vi "editDialog.vi"(0 "reference":refnum<class "CallEdge.lvclass">, 5 "error in (no error)":errorcluster) -> (14 "reference out":refnum<class "CallEdge.lvclass">, 15 "cancel":bool, 19 "error out":errorcluster)   [LabVIEW 2016, in "CallEdge.lvclass"]
doc: "Edit Dialog"
uses:
  <resource>/Framework/Providers/Open_GDS/UML/CallEdge_class/CallEdge.lvclass
  C:/Program Files (x86)/National Instruments/LabVIEW 2016/resource/Framework/Providers/Open_GDS/UML/SegmentedLineEdge_class/SegmentedLineEdge.lvclass
  <resource>/Framework/Providers/Open_GDS/UML/ContextHelp/ContextHelp_HelpTexts.ctl
  <resource>/Framework/Providers/Open_GDS/UML/SegmentedLineEdge_class/SegmentedLineEdge.lvclass
panel:
  in  "OK Button":bool
  in  "Cancel Button":bool
  in  "Help":bool
  in  "Call text":string
  in  "Is signal":bool
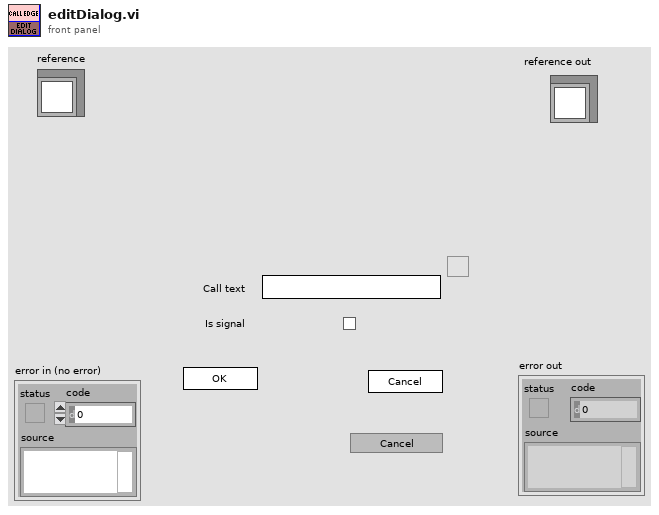
[diagram p1: front panel]
types:
  T1 = typedef "ContextHelp_HelpTexts.ctl" = enum16{"None(Hide)", "Default", "Help", "Welcome", "GettingStarted", "ClassDiagram_Help", "SequenceDiagram_Help", "UseCaseDiagram_Help", "BSelect", "BClass", "BInterface", "BPackage", "BNote", "BDependency", "BInheritance", "BInterfaceImplementation", "BAssociation", "BAggregation", "BCompAggregation", "BNoteConnector", "BObject", "BActionBar", "BCall", "BSystem", "BActor", "BUseCase", "BGeneralization", "BIncludes", "BExtends", "BUseCaseDiagramAssociation", "ClassRelationshipEdge editDialog_Bent Style", "ClassRelationshipEdge editDialog_RelationType", "ClassRelationshipEdge editDialog_Reverse association", "ClassRelationshipEdge editDialog_Start label", "ClassRelationshipEdge editDialog_Middle label", "ClassRelationshipEdge editDialog_End label", "UMLEditor reversedEngineering_Pathes", "ReversedEngineering StateReverseDialog_Help", "ReversedEngineering StateQueuedSettings_Help", "UMLEditor reversedEngineering_AddTopVIs", "UMLEditor reversedEngineering_AddClasses", "UMLEditor reversedEngineering_AddDirs", "UMLEditor reversedEngineering_Recursively", "UMLEditor reversedEngineering_Remove", "UMLEditor reversedEngineering_ClearList", "UMLEditor reversedEngineering_HideSubAss", "UMLEditor reversedEngineering_CreateTypes", "UMLEditor reversedEngineering_OnlyInheritance", "UMLEditor reversedEngineering_CreateApplication", "UMLEditor reversedEngineering_OK", "UMLEditor reversedEngineering_Cancel", "UMLEditor reversedEngineering_Help", "UMLEditor createWizardScriptFile_ScriptfilePath", "UMLEditor createWizardScriptFile_ClassPath", "UMLEditor createWizardScriptFile_Use", "UMLEditor createWizardScriptFile_PrivateDirName", "UMLEditor createWizardScriptFile_DirAppend", "UMLEditor createWizardScriptFile_Separator Character", "UMLEditor createWizardScriptFile_OK", "UMLEditor createWizardScriptFile_Cancel", "UMLEditor createWizardScriptFile_Help", "ClassNode editDialog_Class Name", "InterfaceNode editDialog_Class Name", "ClassNode editDialog_Attribute", "ClassNode editDialog_Methods", "InterfaceNode editDialog_Methods", "ClassNode editDialog_connection", "InterfaceNode editDialog_connection", "ClassNode editDialog_StereoType", "ClassNode editDialog_ShowAttrib", "ClassNode editDialog_ShowMethods", "ClassNode editDialog_ClassPath", "ClassNode editDialog_AddAttribute", "ClassNode editDialog_AddMethod", "InterfaceNode editDialog_AddMethod", "ClassNode AttributeGuide_AttributeName", "ClassNode AttributeGuide_Array?", "ClassNode AttributeGuide_Data Type", "ClassNode AttributeGuide_RefName", "ClassNode AttributeGuide_Preview", "ClassNode AttributeGuide_OK", "ClassNode AttributeGuide_Cancel", "ClassNode MethodGuide_Visibility", "ClassNode MethodGuide_Method Name", "ClassNode MethodGuide_Preview", "ClassNode MethodGuide_OK", "ClassNode MethodGuide_Cancel", "CallNode EditCallProperties_AllButtons", "ObjectNode EditObjectlProperties_AllButtons", "ActorNode EditActorProperties_AllButtons", "UseCaseRelationshipNode EditUseCaselProperties_AllButtons", "UseCaseNode EditUseCaselProperties_AllButtons", "SystemNode EditSystemProperties_AllButtons", "ReversedEngineering UpdateAttributes_AllButtons", "StateNode editDialog_AllButtons", "StateTransition editDialog_AllButtons", "ArrangeNodes Main_Picture", "ArrangeNodes Main_Zoom", "ArrangeNodes Main_Auto Zoom", "ArrangeNodes Main_shorten", "ArrangeNodes Main_Min Length", "ArrangeNodes Main_Max Length", "ArrangeNodes Main_increase", "ArrangeNodes Main_decrease", "ArrangeNodes Main_Shake", "ArrangeNodes Main", "BState", "BInitialState", "BFinalState", "BStateTransition", "StateDiagram_Help", "StateDiagram_PropertiesAllButtons", "ReversedEngineering StateReverseDialog_ClearStates", "ReversedEngineering StateReverseDialog_UseQueuedStateMachines", "ReversedEngineering StateReverseDialog_QueuedSettings", "ReversedEngineering StateReverseDialog_SearchForVIs", "ReversedEngineering StateReverseDialog_SearchCriteria", "OptionsDialog_ClassBasePath", "OptionsDialog_VIPath", "OptionsDialog_ApplicationPath", "OptionsDialog_WizDir", "OptionsDialog_IniFilePath", "OptionsDialog_DefineColors", "OptionsDialog_Help", "OptionsDialog_CreateTypes", "ClassRelationshipEdge editDialog_SplitWire"}
  T2 = typedef "CallEdge.lvclass/ObjectAttributes.ctl" = cluster{"signal":bool}
  T3 = typedef "SegmentedLineEdge.lvclass/ObjectAttributes.ctl" = cluster{"lineStyle":refnum<class "LineStyle.lvclass">, "startArrowHead":refnum<class "ArrowHead.lvclass">, "endArrowHead":refnum<class "ArrowHead.lvclass">, "startLabel":string, "midLabel":string, "endLabel":string, "MidLabelOffset":T4, "SplitWire":bool}
  T4 = typedef "Point Point2D.ctl" = cluster{"x":dbl, "y":dbl}
  T5 = typedef "ContextHelp_ShowType.ctl" = cluster{"Header":string, "Picture":picture, "Text":string}
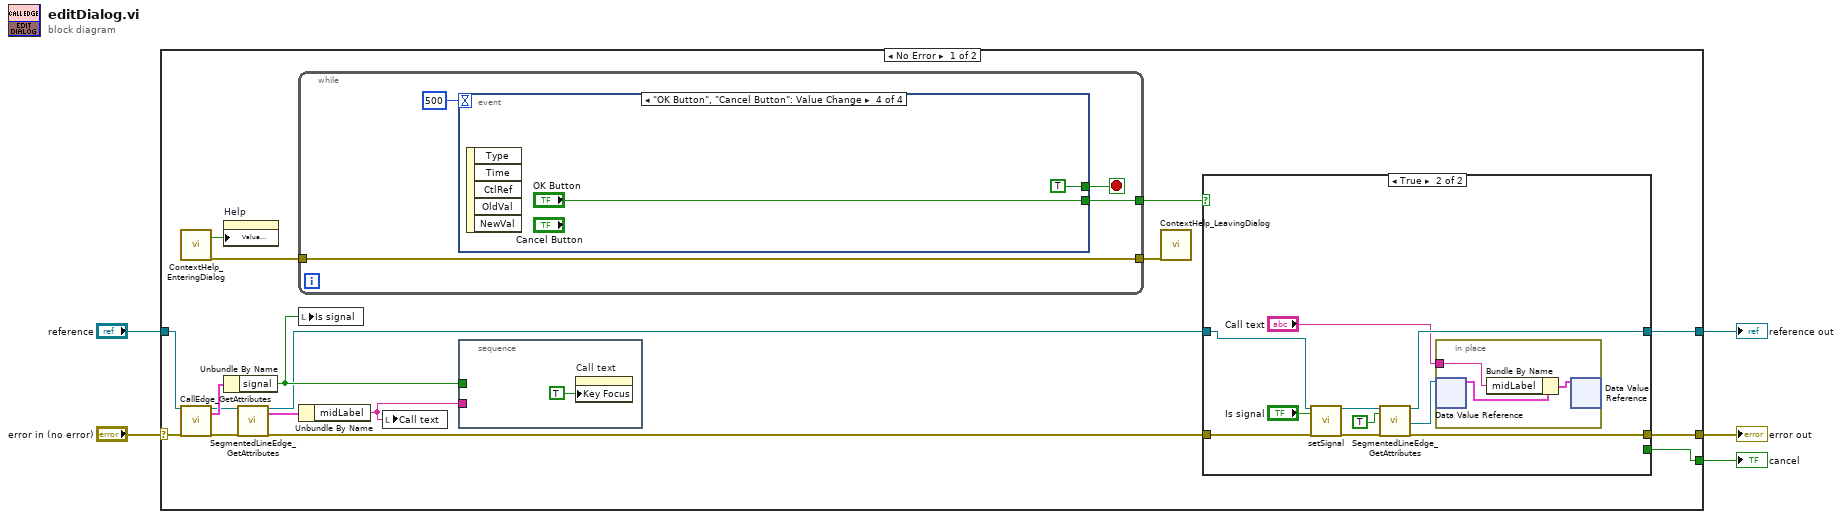
[diagram p0: block diagram]
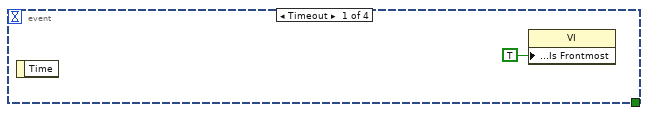
[diagram p2: hidden frame]
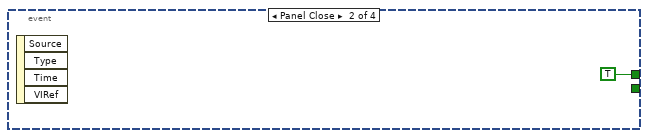
[diagram p3: hidden frame]
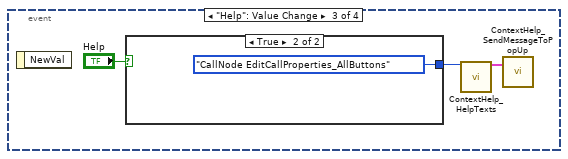
[diagram p4: hidden frame]
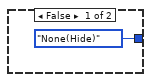
[diagram p5: hidden frame]
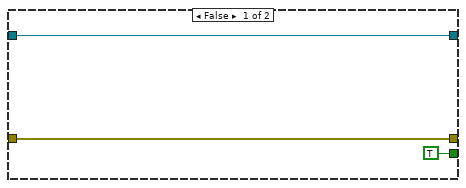
[diagram p6: hidden frame]
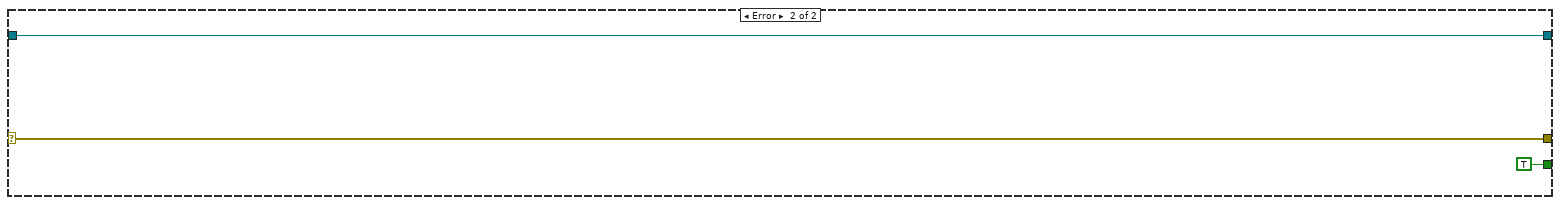
[diagram p7: hidden frame]
diagram:
  n1 = case shown="No Error" "error in (no error)" {
    selector: "error in (no error)" -> [w19 w54]
    tunnel: "reference" -> [w20 w55]
    tunnel: [w22 w54] -> w3
    tunnel: [w21 w55] -> w2
    tunnel: [w18 TRUE ("Key Focus")] -> w1
    frame No Error {
      n2 = call <resource>:"ContextHelp_EnteringDialog.vi"() -> ("HelpStatus"=w13:bool, "error out"=w14:errorcluster)  [unwired: 3 in, 15 out]
      n3 = call <resource>:"CallEdge_GetAttributes.vi"("reference in"=w20, "error in (no error)"=w19) -> ("reference out"=w10:refnum<class "CallEdge.lvclass">, "Data"=w11:T2, "error out"=w9:errorcluster)  [unwired: 1 in, 14 out]
      n4 = property on="Help" class="Bool (strict)"("Value (Signaling)"=w13) -> ()  [unwired: 2 in, 2 out]
      n5 = Unbundle By Name(w11) -> ("signal"=w17:bool)
      n6 = call <resource>:"SegmentedLineEdge_GetAttributes.vi"("reference in"=w10, "error in (no error)"=w9) -> ("reference out"=w7:refnum<class "CallEdge.lvclass">, "Data"=w6:T3, "error out"=w8:errorcluster)  [unwired: 14 in, 1 out]
      n7 = while {
        tunnel: [w26] -> w12
        tunnel: [w24] -> w15
        tunnel: w14 -> [w24]
        stop <- w25 stop-if-true
        n8 = event shown="[3] \"OK Button\", \"Cancel Button\": Value Change" {
          selector: _ -> [_ _ _ _]
          dyn-events: _ -> [_ _ _ _]
          timeout: 500 -> [_ _ _ _]
          tunnel: [_ _ _ "OK Button"] -> w26
          tunnel: [_ TRUE _ TRUE] -> w25
          event Timeout {
            n9 = event-data() -> ()  [unwired: 2 out]
            n10 = property class="VI"("Front Panel Window:Is Frontmost"=TRUE) -> ()  [unwired: 2 in, 2 out]
          }
          event Panel Close {
            n11 = event-data() -> ()  [unwired: 5 out]
          }
          event "Help": Value Change {
            n12 = event-data() -> ()  [unwired: 2 out]
            n13 = case shown="True" "Help" {
              tunnel: [ContextHelp_HelpTexts."None(Hide)" ("HelpText") ContextHelp_HelpTexts."CallNode EditCallProperties_AllButtons" ("HelpText")] -> w30
              frame False {
              }
              frame True {
              }
            }
            n14 = call <resource>:"ContextHelp_HelpTexts.vi"("HelpText (enum or string)"=w30) -> ("HelpOut"=w31:T5)  [unwired: 18 out]
            n15 = call <resource>:"ContextHelp_SendMessageToPopUp.vi"("PopUpMessage"=w31) -> ()  [unwired: 2 in, 17 out]
          }
          event "OK Button", "Cancel Button": Value Change {
            n16 = event-data() -> ()  [unwired: 6 out]
          }
        }
      }
      n17 = local write "Is signal"(w17) -> ()
      n18 = Unbundle By Name(w6) -> ("midLabel"=w16:string)
      n19 = local write "Call text"(w16) -> ()
      n20 = stacked-sequence {
        tunnel: w17 -> [_]
        tunnel: w16 -> [_]
        frame #0 {
          n21 = property on="Call text" class="Str"("Key Focus"=TRUE) -> ()  [unwired: 2 in, 2 out]
        }
      }
      n22 = call <resource>:"ContextHelp_LeavingDialog.vi"("error in (no error)"=w15) -> ()  [unwired: 2 in, 17 out]
      n23 = case shown="True" w12 {
        tunnel: [w36 w48] -> w22
        tunnel: [w38 w47] -> w21
        tunnel: w7 -> [w38 w44]
        tunnel: [TRUE ("Key Focus") _] -> w18
        tunnel: w8 -> [w36 w43]
        frame False {
        }
        frame True {
          n24 = call-dynamic "setSignal.vi"("reference"=w44, "signal"="Is signal", "error in (no error)"=w43) -> ("reference out"=w46:refnum<class "CallEdge.lvclass">, "error out"=w45:errorcluster)  [unwired: 15 out]
          n25 = call <resource>:"SegmentedLineEdge_GetAttributes.vi"("reference in"=w46, "OnlyGetDvrReference(False)"=TRUE, "error in (no error)"=w45) -> ("reference out"=w47:refnum<class "CallEdge.lvclass">, "DataRef"=w40:refnum<data-value>, "error out"=w48:errorcluster)  [unwired: 13 in, 1 out]
          n26 = in-place {
            in-place-border: "Call text" -> [w50]
            n27 = in-place-dvr #1(w40) -> (w51:T3)  [unwired: 1 out]
            n28 = Bundle By Name(cluster=w51, "midLabel"=w50) -> (w49:T3)
            n29 = in-place-dvr #1(w49) -> ()  [unwired: 2 out]
          }
        }
      }
    }
    frame Error {
    }
  }
  "reference out" <- w2
  "error out" <- w3
  "cancel" <- w1
